vi "hind brain 1.vi"() -> ()   [LabVIEW 2011]
uses:
  <vilib>/NXT/Block Support/HWPage.SensorType.ctl
  <vilib>/NXT/Block Support/HWPage.SensorMode.ctl
  <vilib>/NXT/Block Support/NXT_InputPort.ctl
  <vilib>/NXT/Dual Mode Library/Sensors/Color_None.vi
  New Sensors/mindsensors.com_LVEE_Toolkit/mindsensors.com_LVEE_Toolkit_V1.23/mindsensors.com LVEE Toolkit/Dual/NXTServo-DM.vi
panel:
  in  "SERVO 2 SPEED":u8(slide) step=1 scale=0.0..255.0
  in  "SERVO 2 POSITION":u16(slide)=1500 min=500 max=2500 scale=500.0..2500.0
  in  "stop 2":bool
  out "Output Servo  TWO":cluster{"Voltage":u8, "Status":bool}
  in  "SERVO 1 POSITION":u16(slide)=1500 min=500 max=2500 scale=500.0..2500.0
  in  "SERVO 1 SPEED":u8(slide) step=1 scale=0.0..255.0
  out "Pressed?":bool caption="Switch\nPressed?"
  out "Light Intensity":i16 caption="Scaled Value"
  out "Battery mv":i32
  out "Blink":bool
  out "Scaled Value":i16
  out "Left?":bool
  out "Right?":bool
  out "Front?":bool
  out "Stuff?":bool
  in  "stop":bool
  out "Output Servo ONE":cluster{"Voltage":u8, "Status":bool}
  # "This is a demonstration of how to sense and acturate devices on the LEGO NXT brick.\nThe connections to the NXT brick are as follows:\nNOTHING IS CONNECTED TO PORTS A, B AND C.\nPort 1 has the Mindsensor NXTServo\nPort 2 has the LEGO Color Sensor\nPort 3 has the LEGO Switch\nPort 4 and the Mindsensor NXTSumoEyes-v3."
  # "SENSORS"
  # "ACTUATORS"
  # "SUMO SENSOR"
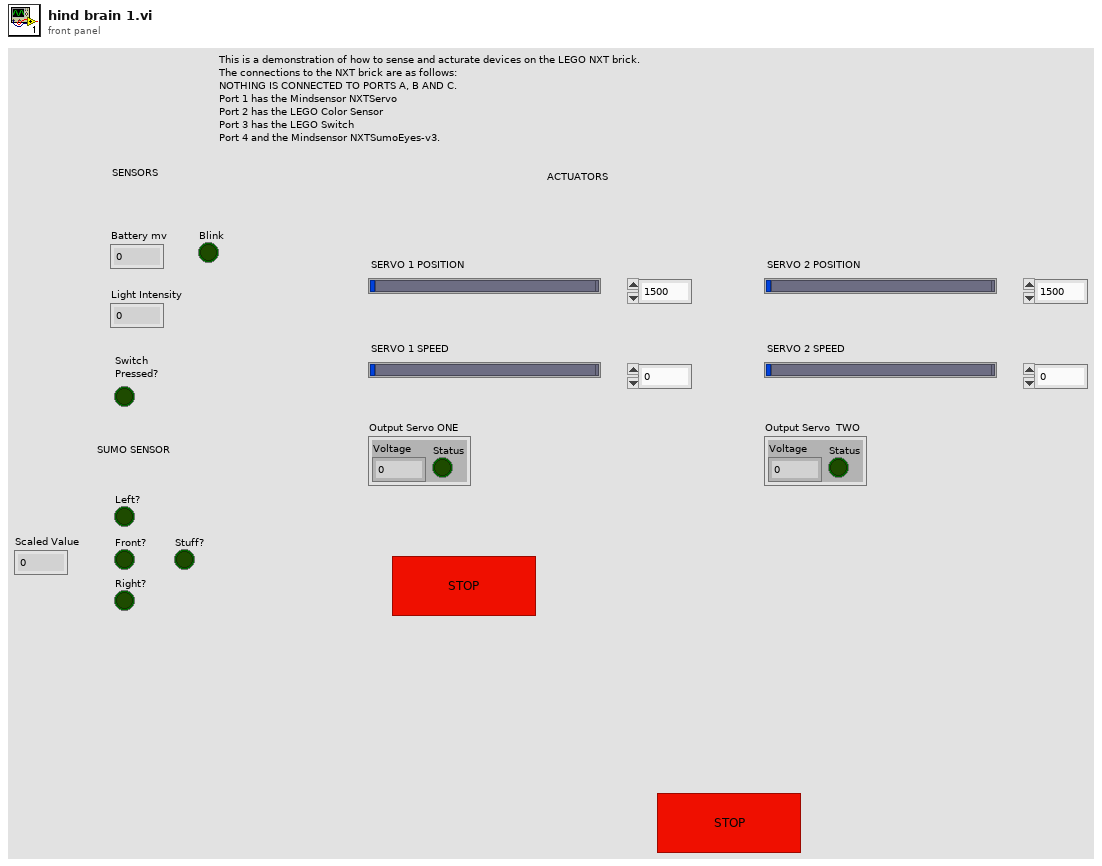
[diagram p1: front panel]
types:
  T1 = cluster{"Servo Number":u8, "Position":u16, "Speed":u8}
  T2 = typedef "NXT_InputPort.ctl" = u8
  T3 = typedef "HWPage.SensorType.ctl" = u8
  T4 = typedef "HWPage.SensorMode.ctl" = u8
  T5 = typedef "LVHSConnector.ctl" = cluster{"Hardware":string, "Flattened String":string}
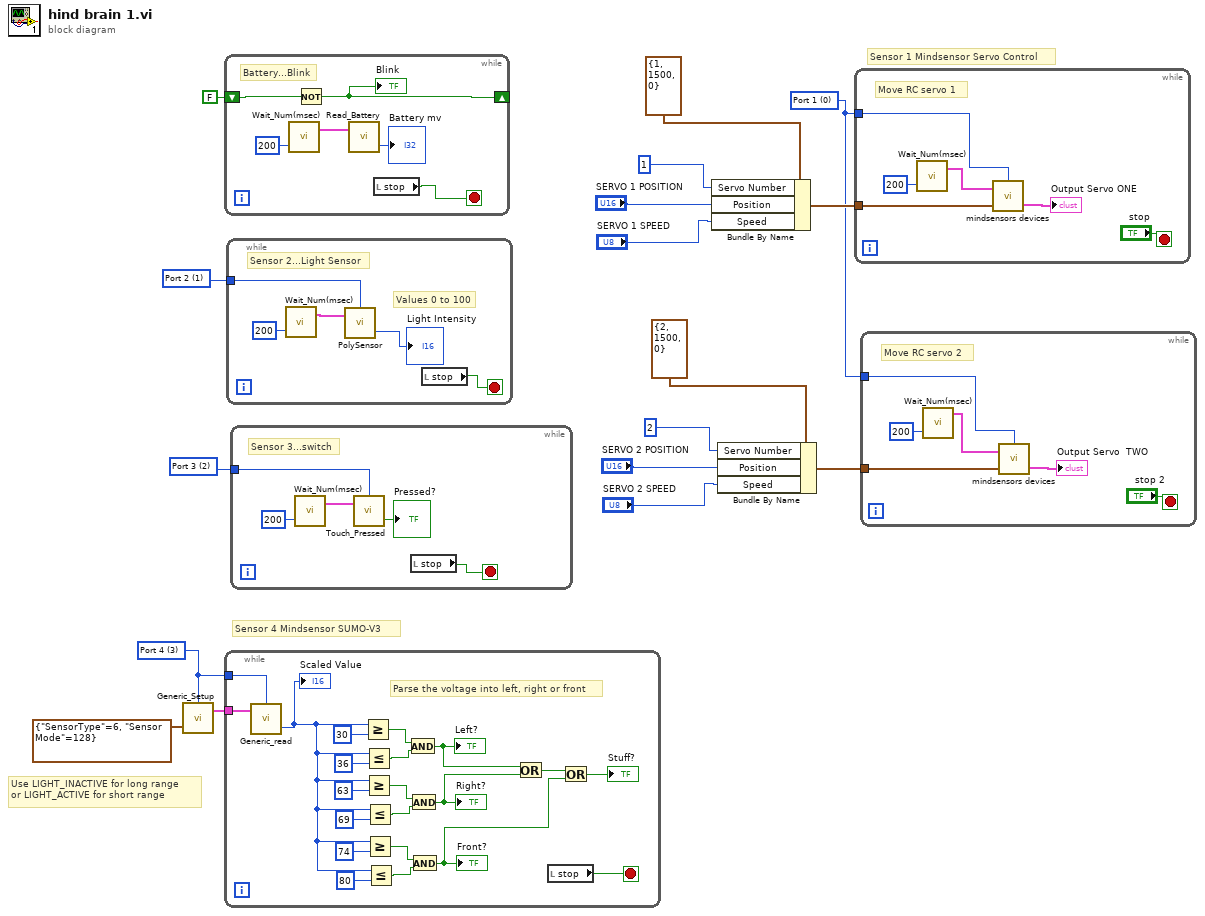
[diagram p0: block diagram]
diagram:
  w12 = T2 2 items=["Port 1", "Port 2", "Port 3", "Port 4"] ("Port (Port 1)")
  w13 = T2 1 items=["Port 1", "Port 2", "Port 3", "Port 4"] ("Port (Port 3)")
  w1 = T2 0 items=["Port 1", "Port 2", "Port 3", "Port 4"] ("Input Port")
  w14 = T2 3 items=["Port 1", "Port 2", "Port 3", "Port 4"] ("Port")
  # "Sensor 4 Mindsensor SUMO-V3"
  # "Sensor 1 Mindsensor Servo Control"
  # "Use LIGHT_INACTIVE for long range\nor LIGHT_ACTIVE for short range"
  n1 = call <vilib>:"Generic_Setup.vi"("Sensor Setup"=cluster{"SensorType":T3, "Sensor Mode":T4} {"SensorType"=6, "Sensor Mode"=128}, "Port"=w14) -> ("NXT"=w17:T5)  [unwired: 1 in, 1 out]
  n2 = while {
    shift-right: [w19] -> _
    shift-left: FALSE -> [w20]
    stop <- w21 stop-if-true
    # "Battery...Blink"
    n3 = call <vilib>:"Wait_Num(msec).vi"("Time (100 msec)"=u32 200) -> ("NXT"=w22:T5)  [unwired: 3 in]
    n4 = Not(x=w20) -> (.not. x?=w19:bool)
    "Blink" <- w19
    n5 = call <vilib>:"Read_Battery.vi"("NXT"=w22) -> ("millivolts"=→"Battery mv":i32)  [unwired: 2 in, 1 out]
    n6 = local read "stop"() -> (w21:bool)
  }
  n7 = while {
    tunnel: w14 -> [w44]
    tunnel: w17 -> [w43]
    stop <- w24 stop-if-true
    # "Parse the voltage into left, right or front"
    n8 = call <vilib>:"Generic_read.vi"("NXT"=w43, "Port (Port 3)"=w44) -> ("Scaled Value"=w30:i16)  [unwired: 2 out]
    "Scaled Value" <- w30
    n9 = Greater Or Equal?(x=w30, y=i16 30) -> (x >= y?=w40:bool)
    n10 = Less Or Equal?(x=w30, y=i16 36) -> (x <= y?=w39:bool)
    n11 = Greater Or Equal?(x=w30, y=i16 63) -> (x >= y?=w37:bool)
    n12 = Less Or Equal?(x=w30, y=i16 69) -> (x <= y?=w38:bool)
    n13 = Greater Or Equal?(x=w30, y=i16 74) -> (x >= y?=w33:bool)
    n14 = Less Or Equal?(x=w30, y=i16 80) -> (x <= y?=w34:bool)
    n15 = And(x=w40, y=w39) -> (x .and. y?=w29:bool)
    "Left?" <- w29
    n16 = And(x=w37, y=w38) -> (x .and. y?=w28:bool)
    "Right?" <- w28
    n17 = And(x=w33, y=w34) -> (x .and. y?=w26:bool)
    "Front?" <- w26
    n18 = Or(x=w29, y=w28) -> (x .or. y?=w27:bool)
    n19 = local read "stop"() -> (w24:bool)
    n20 = Or(x=w27, y=w26) -> (x .or. y?=→"Stuff?":bool)
  }
  n21 = while {
    tunnel: w13 -> [w45]
    stop <- w48 stop-if-true
    # "Values 0 to 100"
    # "Sensor 2...Light Sensor"
    n22 = call <vilib>:"Wait_Num(msec).vi"("Time (100 msec)"=u32 200) -> ("NXT"=w47:T5)  [unwired: 3 in]
    n23 = call-poly <vilib>:"PolySensor.vi"("NXT"=w47, "Port (Port 3)"=w45) -> ("Intensity"=→"Light Intensity":i16)  [unwired: 1 in, 1 out]
    n24 = local read "stop"() -> (w48:bool)
  }
  n25 = while {
    tunnel: w12 -> [w51]
    stop <- w52 stop-if-true
    # "Sensor 3...switch"
    n26 = call <vilib>:"Wait_Num(msec).vi"("Time (100 msec)"=u32 200) -> ("NXT"=w53:T5)  [unwired: 3 in]
    n27 = call <vilib>:"Touch_Pressed.vi"("NXT"=w53, "Port (Port 1)"=w51) -> ("Yes / No"=→"Pressed?":bool)  [unwired: 1 in, 1 out]
    n28 = local read "stop"() -> (w52:bool)
  }
  n29 = Bundle By Name(cluster=T1 {"Servo Number"=1, "Position"=1500, "Speed"=0} ("Input of NXTServo"), "Servo Number"=u8 1, "Position"="SERVO 1 POSITION", "Speed"="SERVO 1 SPEED") -> (w10:T1)
  n30 = Bundle By Name(cluster=T1 {"Servo Number"=2, "Position"=1500, "Speed"=0} ("Input of NXTServo"), "Servo Number"=u8 2, "Position"="SERVO 2 POSITION", "Speed"="SERVO 2 SPEED") -> (w5:T1)
  n31 = while {
    tunnel: w1 -> [w58]
    tunnel: w10 -> [w57]
    stop <- "stop" stop-if-true
    # "Move RC servo 1"
    n32 = call <vilib>:"Wait_Num(msec).vi"("Time (100 msec)"=u32 200) -> ("NXT"=w55:T5)  [unwired: 3 in]
    n33 = call-poly "mindsensors devices.vi"("Input of NXTServo"=w57, "NXT"=w55, "Input Port"=w58) -> ("Output of NXTServo"=→"Output Servo ONE":cluster{"Voltage":u8, "Status":bool})  [unwired: 1 out]
  }
  n34 = while {
    tunnel: w1 -> [w64]
    tunnel: w5 -> [w63]
    stop <- "stop 2" stop-if-true
    # "Move RC servo 2"
    n35 = call <vilib>:"Wait_Num(msec).vi"("Time (100 msec)"=u32 200) -> ("NXT"=w61:T5)  [unwired: 3 in]
    n36 = call-poly "mindsensors devices.vi"("Input of NXTServo"=w63, "NXT"=w61, "Input Port"=w64) -> ("Output of NXTServo"=→"Output Servo  TWO":cluster{"Voltage":u8, "Status":bool})  [unwired: 1 out]
  }
